vi "WebDAV_Direcctory_Listings.vi"() -> ()   [LabVIEW 2014]
uses:
  <vilib>/WebDAVClient/NI_WebDAV.lvlib
panel:
  in  "relative uri":string="files/ni-rt/startup/sample/"
  in  "host uri prefix":string="http://169.254.254.10/"
  in  "Listbox":i32(listbox)
  in  "error in (no error)":errorcluster
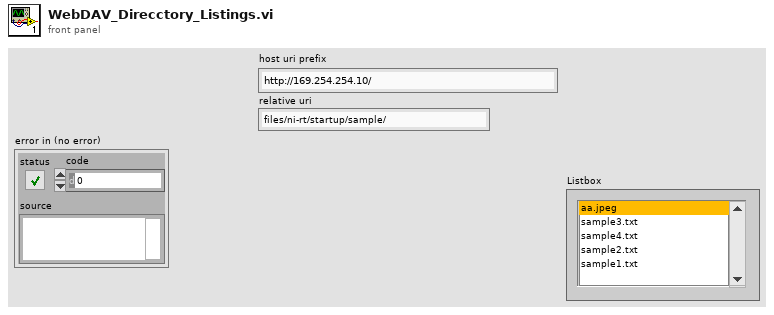
[diagram p1: front panel]
types:
  T1 = typedef "NI_WebDAV.lvlib/SessionHandle.ctl" = refnum<k1>
  T2 = typedef "NI_WebDAV.lvlib/FileInfo.ctl" = cluster{"type":string, "size":u64, "last modification":timestamp, "display name":string, "uri":string}
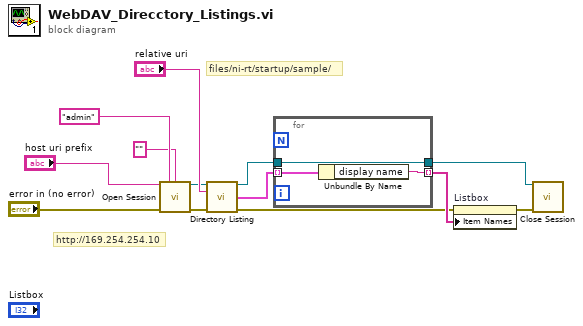
[diagram p0: block diagram]
diagram:
  # "files/ni-rt/startup/sample/"
  # "http://169.254.254.10"
  n1 = call <vilib>:"Open Session.vi"("host uri prefix"="host uri prefix", "username"="admin", "password"="", "error in (no error)"="error in (no error)") -> ("session handle out"=w7:T1, "error out"=w10:errorcluster)  [unwired: 10 in]
  n2 = call <vilib>:"Directory Listing.vi"("session handle"=w7, "relative uri"="relative uri", "error in (no error)"=w10) -> ("session handle out"=w3:T1, "file list"=w12:T2[], "error out"=w5:errorcluster)  [unwired: 9 in, 1 out]
  n3 = for {
    tunnel: w12 -> [w16] mode=indexing
    tunnel: [w15] -> w11 mode=indexing
    tunnel: [w14] -> w4
    tunnel: w3 -> [w14]
    n4 = Unbundle By Name(w16) -> ("display name"=w15:string)
  }
  n5 = property on="Listbox" class="LstBox (strict)"(error in=w5, "Item Names"=w11) -> (error out=w6:errorcluster)  [unwired: 1 in, 1 out]
  n6 = call <vilib>:"Close Session.vi"("session handle"=w4, "error in (no error)"=w6) -> ()  [unwired: 13 in, 1 out]
